vi "Write to Hardware.vi"(7 "Valid Triggers":bool, 8 "error in":errorcluster, 9 "Trigger Values":dbl[](array[numeric]), 10 "Values in":dbl[](array[numeric]), 11 "Tx UDP Execution Unit in":refnum<class "Tx UDP Execution Unit.lvclass">) -> (0 "error out":errorcluster, 1 "Trigger Values out":dbl[](array[numeric]), 2 "Values out":dbl[](array[numeric]), 3 "Tx UDP Execution Unit out":refnum<class "Tx UDP Execution Unit.lvclass">)   [LabVIEW 2020, in "AIM ARINC 664 Engine.lvlib" / "Implementation.lvlib" / "Tx UDP Execution Unit.lvclass"]
uses:
  Tx UDP Execution Unit.lvclass
  Tx UDP Execution Unit.lvclass/Tx UDP Execution Unit.ctl
  <vilib>/Utility/SystemLogging/NI_SystemLogging.lvlib
  <instrlib>/AIM GmbH/_AIM 664/AIM664LV.lvlib
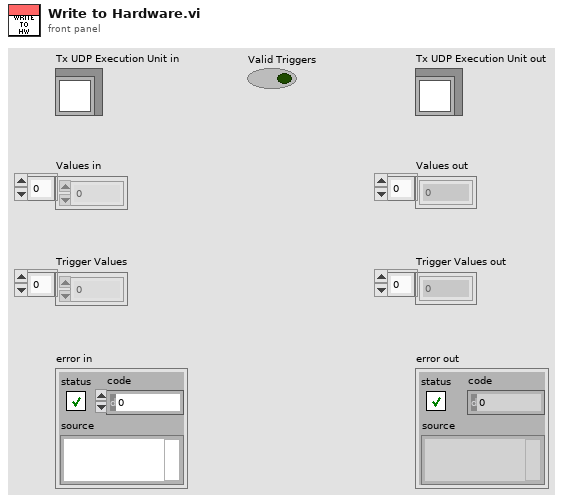
[diagram p1: front panel]
types:
  T1 = typedef "Encoding (Arinc664).ctl" = u16
  T2 = cluster{"Data":u8[], "Parameters":cluster{"start index":i32, "size":i32, "encoding":T1, "signed":bool, "scale multiplier":dbl, "scale offset":dbl}[]}[]
  T3 = cluster{"Data":u8[], "Parameters":cluster{"start index":i32, "size":i32, "encoding":T1, "signed":bool, "scale multiplier":dbl, "scale offset":dbl}[]}
  T4 = cluster{"start index":i32, "size":i32, "encoding":T1, "signed":bool, "scale multiplier":dbl, "scale offset":dbl}[]
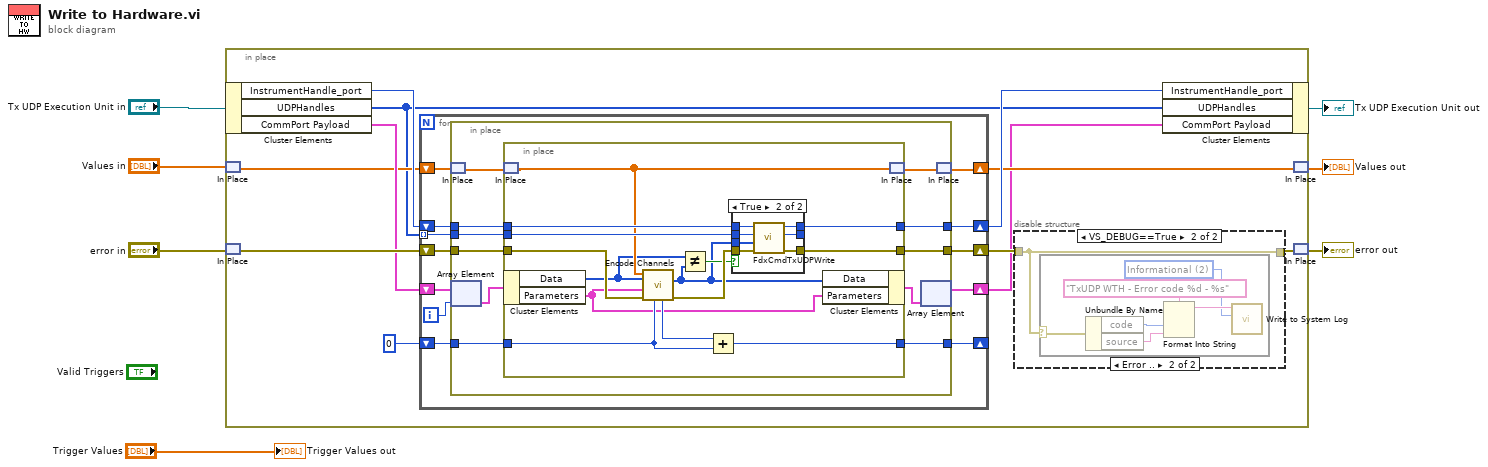
[diagram p0: block diagram]
diagram:
  n1 = in-place {
    n2 = in-place-cluster #1("Tx UDP Execution Unit in") -> ("InstrumentHandle_port"=w18:u32, "UDPHandles"=w9:u32[], "CommPort Payload"=w15:T2)
    n3 = in-place-match #2("Values in") -> (w14:dbl[])
    n4 = in-place-match #3("error in") -> (w17:errorcluster)
    n5 = for {
      tunnel: w9 -> [w37] mode=indexing
      shift-right: [w35] -> w16
      shift-left: w18 -> [w38]
      shift-right: [w36] -> w13
      shift-left: w17 -> [w34]
      shift-right: [w32] -> _
      shift-left: 0 -> [w33]
      shift-right: [w28] -> w10
      shift-left: w14 -> [w29]
      shift-right: [w27] -> w8
      shift-left: w15 -> [w31]
      i -> [w30]
      n6 = in-place {
        in-place-border: w38 -> [w49]
        in-place-border: w37 -> [w48]
        in-place-border: [w47] -> w36
        in-place-border: [w46] -> w35
        in-place-border: w34 -> [w45]
        in-place-border: w33 -> [w44]
        in-place-border: [w43] -> w32
        n7 = in-place-match #4(w29) -> (w41:dbl[])
        n8 = in-place-array #5(w31, w30) -> (w42:T3)
        n9 = in-place {
          in-place-border: w49 -> [w63]
          in-place-border: w48 -> [w62]
          in-place-border: [w61] -> w47
          in-place-border: [w60] -> w46
          in-place-border: w45 -> [w59]
          in-place-border: w44 -> [w56]
          in-place-border: [w55] -> w43
          n10 = in-place-match #6(w41) -> (w54:dbl[])
          n11 = in-place-cluster #7(w42) -> ("Data"=w52:u8[], "Parameters"=w53:T4)
          n12 = call "Encode Channels.vi"("Offset"=w56, "error in"=w59, "Parameters"=w53, "Data in"=w52, "Values in"=w54) -> ("error out"=w58:errorcluster, "Data out"=w50:u8[], "Number of Parameters"=w57:i32)  [unwired: 4 in]
          n13 = Not Equal?(x=w52, y=w50) -> (x != y?=w51:bool)
          n14 = Add(x=w57, y=w56) -> (x+y=w55:i32)
          n15 = case shown="True" w51 {
            tunnel: w63 -> [w66 w73]
            tunnel: w62 -> [w65 w72]
            tunnel: [w64 w71] -> w61
            tunnel: [w66 w70] -> w60
            tunnel: [w65 w69] -> _
            tunnel: w58 -> [w64 w68]
            tunnel: w50 -> [_ w67]
            frame False {
            }
            frame True {
              n16 = call <instrlib>:"FdxCmdTxUDPWrite.vi"("error in"=w68, "Data"=w67, "UdpHandle"=w72, "InstrumentHandle"=w73) -> ("error out"=w71:errorcluster, "UdpHandleOut"=w69:u32, "InstrumentHandle"=w70:u32)  [unwired: 4 in, 1 out]
            }
          }
          n17 = in-place-cluster #7("Data"=w50, "Parameters"=w53) -> (w39:T3)
          n18 = in-place-match #6(w54) -> (w40:dbl[])
        }
        n19 = in-place-array #5(w39) -> (w27:T2)  [unwired: 1 out]
        n20 = in-place-match #4(w40) -> (w28:dbl[])
      }
    }
    n21 = disable-structure shown="VS_DEBUG==True" {
      disable-tunnel: w13 -> [w19 w20]
      disable-tunnel: [w19 w20] -> w12
      frame condition #0 (active) {
      }
      frame condition #1 {
        n22 = case shown="Error .." w20 {
          selector: w20 -> [_ w21]
          frame No Error {
          }
          frame Error {
            w24 = 2 items=["Error", "Warning", "Informational"] ("severity")
            n23 = Unbundle By Name(w21) -> ("code"=w23:i32, "source"=w22:string)
            n24 = Format Into String(format string="TxUDP WTH - Error code %d - %s", w23, w22) -> (resulting string=w25:string)  [unwired: 2 in, 1 out]
            n25 = call <vilib>:"Write to System Log.vi"("severity"=w24, "message"=w25) -> ()  [unwired: 9 in, 1 out]
          }
        }
      }
    }
    n26 = in-place-cluster #1("InstrumentHandle_port"=w16, "UDPHandles"=w9, "CommPort Payload"=w8) -> (→"Tx UDP Execution Unit out":refnum<class "Tx UDP Execution Unit.lvclass">)
    n27 = in-place-match #2(w10) -> (→"Values out":dbl[])
    n28 = in-place-match #3(w12) -> (→"error out":errorcluster)
  }
  "Trigger Values out" <- "Trigger Values"
